vi "MatlabControlBindingTest.vi"() -> ()   [LabVIEW 2017]
uses:
  Types/ControlValueChangeEventBindingType.ctl
panel:
  out "Changed Control name":string
  out "Changed control new value":variant
  in  "ExpID":string
  in  "Boolean":bool
  in  "String":string
  in  "Numeric":dbl
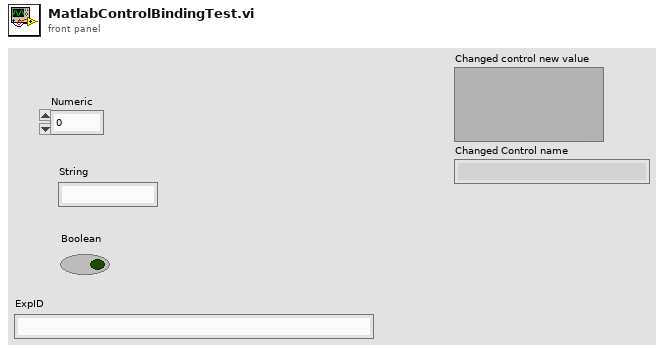
[diagram p1: front panel]
types:
  T1 = typedef "ControlValueChangeEventBindingType.ctl" = cluster{"Control":refnum<vi>, "Event Register":refnum<event-registration>}
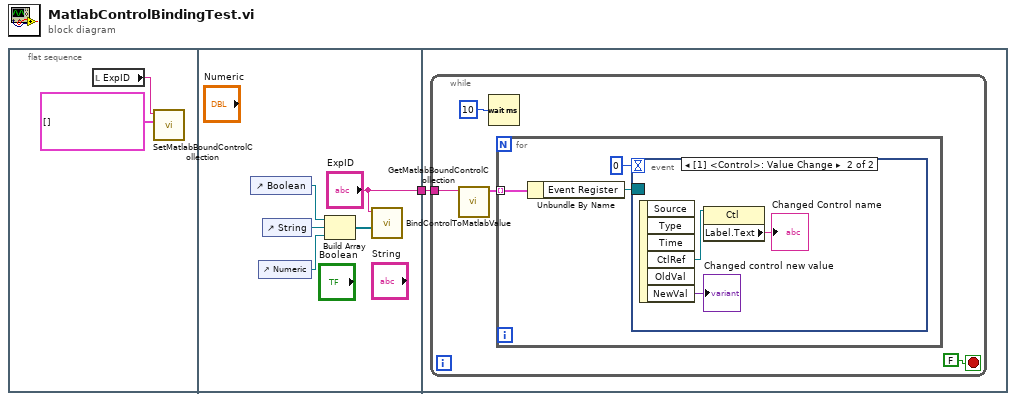
[diagram p0: block diagram]
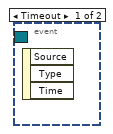
[diagram p2: hidden frame]
diagram:
  n1 = flat-sequence {
    tunnel: ["ExpID"] -> w1
    tunnel: w1 -> [w9]
    frame #0 {
      n2 = local read "ExpID"() -> (w2:string)
      n3 = call "SetMatlabBoundControlCollection.vi"("Bound controls"=T1[] [], "ExpID"=w2) -> ()  [unwired: 10 in]
    }
    frame #1 {
      n4 = control-ref of="Boolean"() -> (w8:refnum<vi>)
      n5 = control-ref of="Numeric"() -> (w6:refnum<vi>)
      n6 = control-ref of="String"() -> (w7:refnum<vi>)
      n7 = Build Array(w8, w7, w6) -> (w5:refnum<vi>[])
      n8 = call "BindControlToMatlabValue.vi"("Controls[]"=w5, "ExpID"="ExpID") -> ()  [unwired: 9 in, 1 out]
    }
    frame #2 {
      n9 = while {
        tunnel: w9 -> [w10]
        stop <- FALSE stop-if-true
        n10 = call "GetMatlabBoundControlCollection.vi"("ExpID"=w10) -> ("Bound Controls"=w12:T1[])  [unwired: 10 in]
        n11 = Wait (ms)(milliseconds to wait=u32 10) -> ()  [unwired: 1 out]
        n12 = for {
          tunnel: w12 -> [w16] mode=indexing
          n13 = Unbundle By Name(w16) -> ("Event Register"=w15:refnum<event-registration>)
          n14 = event shown="[1] <Control>: Value Change" {
            selector: w15 -> [_ _]
            dyn-events: _ -> [_ _]
            timeout: 0 -> [_ _]
            event Timeout {
              n15 = event-data() -> ()  [unwired: 1 in, 3 out]
            }
            event Value Change {
              n16 = event-data() -> ("CtlRef"=w18:refnum<vi>, "NewVal"=→"Changed control new value":variant)  [unwired: 1 in, 4 out]
              n17 = property class="Ctl"(reference=w18) -> ("Label.Text"=→"Changed Control name":string)  [unwired: 1 in, 2 out]
            }
          }
        }
      }
    }
  }
